vi "Test_Copy_Image_Greyscale_Mask_ARGB.vi"(8 "error in (no error)":errorcluster, 11 "Test Case In":refnum<class "Image.lvclass">) -> (0 "error out":errorcluster, 3 "Test Case Out":refnum<class "Image.lvclass">)   [LabVIEW 2020, in "g_ar_toolkit.test.lvlib" / "Image.lvclass"]
uses:
  Image.lvclass
  Image.lvclass/Image.ctl
  g_ar_toolkit.image/g_ar_toolkit.image.lvlib
  g_ar_toolkit.image/Image Size (Fixed).ctl
  g_ar_toolkit.image/CopyImageGreyscaleMaskARGB.vi
  g_ar_toolkit.image/CreateEmptyImageGreyscale.vi
  g_ar_toolkit.image/CreateEmptyImageARGB.vi
  g_ar_toolkit.image/ARGB Colour.ctl
  4993e8ee-a06a-463a-9684-69129f64d5ce.vi
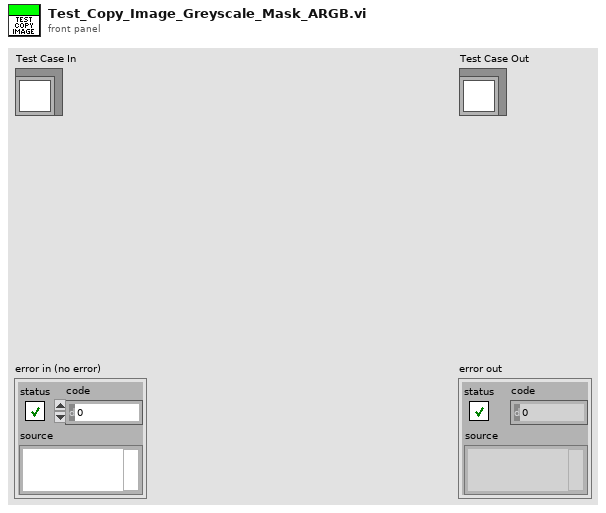
[diagram p1: front panel]
types:
  T1 = typedef "g_ar_toolkit.image.lvlib/ARGB Colour.ctl" = cluster{"Alpha":u8, "RGB":u32}
  T2 = typedef "g_ar_toolkit.image.lvlib/Image Size (Fixed).ctl" = cluster{"Width":u16, "Height":u16}
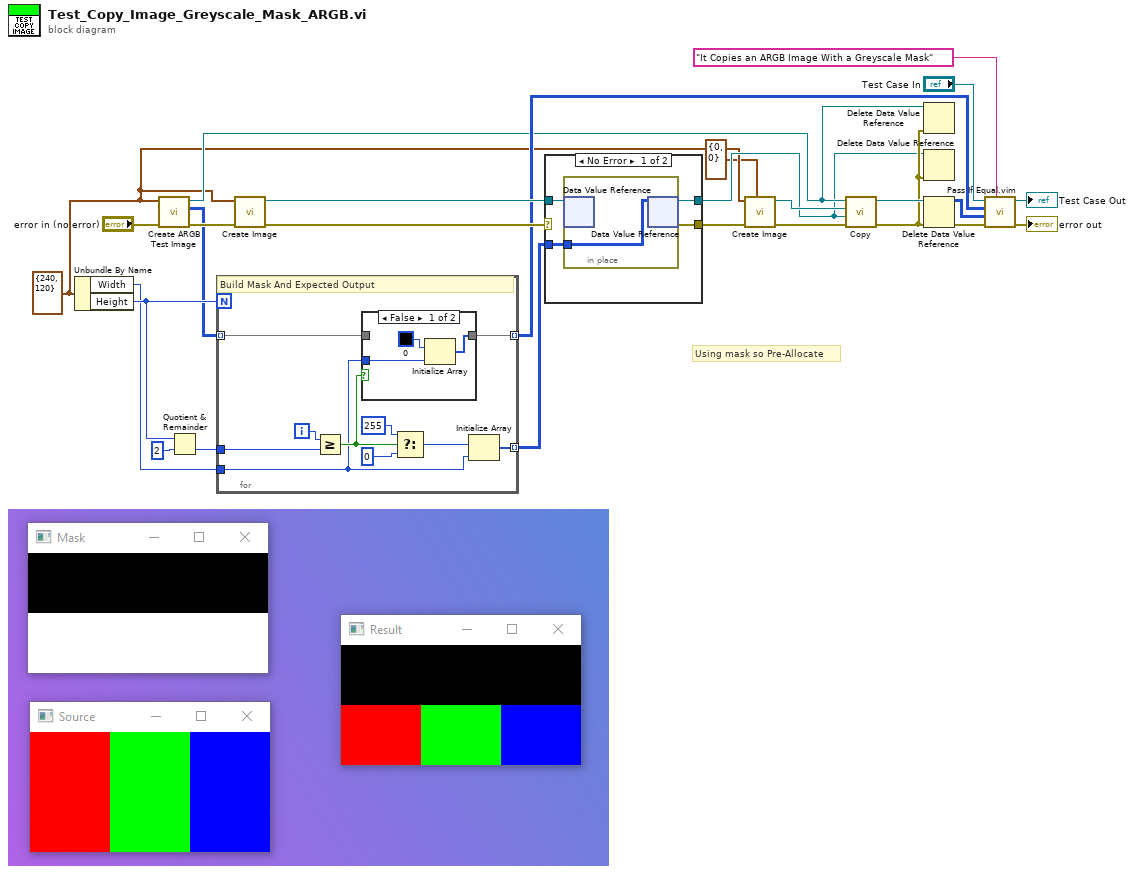
[diagram p0: block diagram]
diagram:
  w2 = T2 {"Width"=240, "Height"=120} ("Preallocated Image Size (Default - 0,0)")
  # "Using mask so Pre-Allocate"
  n1 = Unbundle By Name(w2) -> ("Width"=w13:u16, "Height"=w14:u16)
  n2 = call "Create ARGB Test Image.vi"("error in (no error)"="error in (no error)", "Preallocated Image Size"=w2) -> ("error out"=w8:errorcluster, "24-bit pixmap"=w7:u32[][], "Data Value Reference out"=w4:refnum<data-value>)  [unwired: 7 in]
  n3 = Quotient & Remainder(x=w14, y=u16 2) -> (floor(x/y)=w12:u16)  [unwired: 1 out]
  n4 = for {
    N: w14 -> [_]
    tunnel: [w31] -> w20 mode=indexing
    tunnel: w13 -> [w27]
    tunnel: w12 -> [w35]
    tunnel: w7 -> [w30] mode=indexing
    tunnel: [w28] -> w11 mode=indexing
    i -> [w36]
    # "Build Mask And Expected Output"
    n5 = Greater Or Equal?(x=w36, y=w35) -> (x >= y?=w29:bool)
    n6 = case shown="False" w29 {
      tunnel: w30 -> [_ w40]
      tunnel: [w37 w40] -> w28
      tunnel: w27 -> [w39 _]
      frame False {
        n7 = Initialize Array(u32 0 ("element"), w39) -> (w37:u32[])
      }
      frame True {
      }
    }
    n8 = Select(t=u8 255, s=w29, f=u8 0) -> (s? t:f=w32:u8)
    n9 = Initialize Array(w32, w27) -> (w31:u8[])
  }
  n10 = call-poly "Create Image.vi"("error in (no error)"=w8, "Preallocated Image Size (Default 0,0)"=w2) -> ("error out"=w18:errorcluster, "New Greyscale Image"=w19:refnum<data-value>)  [unwired: 8 in]
  n11 = case shown="No Error" w18 {
    selector: w18 -> [_ w46]
    tunnel: w19 -> [w44 w47]
    tunnel: [w43 w47] -> w3
    tunnel: [w42 w46] -> w16
    tunnel: w20 -> [w41 _]
    frame No Error {
      n12 = in-place {
        in-place-border: w41 -> [w45]
        n13 = in-place-dvr #1(w44) -> ()  [unwired: 2 out]
        n14 = in-place-dvr #1(w45) -> (w43:refnum<data-value>, w42:errorcluster)
      }
    }
    frame Error {
    }
  }
  n15 = call-poly "Create Image.vi"("Colour (Default: Black)"=T1 {"Alpha"=0, "RGB"=0}, "error in (no error)"=w16, "Preallocated Image Size (Default: 0,0)"=w2) -> ("error out"=w22:errorcluster, "New ARGB Image"=w6:refnum<data-value>)  [unwired: 7 in]
  n16 = call-poly "Copy.vi"("error in (no error)"=w22, "Greyscale Image Mask"=w3, "ARGB Image Destination"=w6, "ARGB Image Source"=w4) -> ("error out"=w5:errorcluster, "ARGB Image Destination (duplicate)"=w10:refnum<data-value>)  [unwired: 6 in]
  n17 = Delete Data Value Reference(data value reference=w4, error in=w5) -> ()  [unwired: 2 out]
  n18 = Delete Data Value Reference(data value reference=w3, error in=w5) -> ()  [unwired: 2 out]
  n19 = Delete Data Value Reference(data value reference=w10, error in=w5) -> (data value=w21:u32[][], error out=w17:errorcluster)
  n20 = call "Pass If Equal.vim"("Description"="It Copies an ARGB Image With a Greyscale Mask", "error in (no error)"=w17, "Actual"=w21, "Expected"=w11, "LUnit Test Case In"="Test Case In") -> ("error out"=→"error out":errorcluster, "LUnit Test Case Out"=→"Test Case Out":refnum<class "Image.lvclass">)  [unwired: 5 in]
